vi "writeToLogFile.vi"(0 "Values":dbl[](array[numeric]), 1 "Names":string[](array[string]), 2 "Overwrite?":bool, 3 "File Path":string="C:\\spreadsheet.xls") -> ()   [LabVIEW 2012]
uses:
  <vilib>/Utility/file.llb/Write To Spreadsheet File (string).vi
  <vilib>/Utility/file.llb/Write To Spreadsheet File (DBL).vi
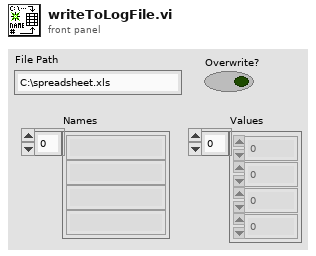
[diagram p1: front panel]
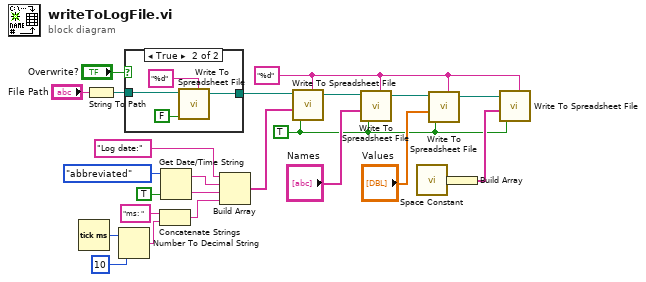
[diagram p0: block diagram]
diagram:
  w8 = "%d" ("format (%.3f)")
  w11 = TRUE
  n1 = Tick Count (ms)() -> (millisecond timer value=w7:u32)
  n2 = String To Path(string="File Path") -> (path=w1:path)
  n3 = Number To Decimal String(number=w7, width (-)=i16 10) -> (decimal integer string=w4:string)
  n4 = case shown="True" "Overwrite?" {
    tunnel: w1 -> [w25 w28]
    tunnel: [w25 w27] -> w9
    frame False {
    }
    frame True {
      n5 = call-poly <vilib>:"Write To Spreadsheet File.vi"("format (%.3f)"="%d", "append to file? (new file:F)"=FALSE, "file path (dialog if empty)"=w28) -> ("new file path (Not A Path if cancelled)"=w27:path)  [unwired: 5 in]
    }
  }
  n6 = Concatenate Strings("ms: " ("string"), w4) -> (w3:string)
  n7 = Get Date/Time String(date format (0)=enum16{"short", "long", "abbreviated"}."abbreviated", want seconds? (F)=TRUE) -> (date string=w18:string, time string=w17:string)  [unwired: 1 in]
  n8 = Build Array("Log date:", w18, w17, w3) -> (w14:string[])
  n9 = call-poly <vilib>:"Write To Spreadsheet File.vi"("format (%s)"=w8, "append to file? (new file:F)"=w11, "1D data"=w14, "file path (dialog if empty)"=w9) -> ("new file path (Not A Path if cancelled)"=w15:path)  [unwired: 4 in]
  n10 = call-poly <vilib>:"Write To Spreadsheet File.vi"("format (%s)"=w8, "append to file? (new file:F)"=w11, "1D data"="Names", "file path (dialog if empty)"=w15) -> ("new file path (Not A Path if cancelled)"=w23:path)  [unwired: 4 in]
  n11 = call <vilib>:"Space Constant.vi"() -> ("String"=w16:string)
  n12 = call-poly <vilib>:"Write To Spreadsheet File.vi"("format (%.3f)"=w8, "append to file? (new file:F)"=w11, "1D data"="Values", "file path (dialog if empty)"=w23) -> ("new file path (Not A Path if cancelled)"=w13:path)  [unwired: 4 in]
  n13 = Build Array(w16) -> (w12:string[])
  n14 = call-poly <vilib>:"Write To Spreadsheet File.vi"("format (%s)"=w8, "append to file? (new file:F)"=w11, "1D data"=w12, "file path (dialog if empty)"=w13) -> ()  [unwired: 4 in, 1 out]
